vi "Definition.vi"(11 "User":refnum<class "User.lvclass">) -> (2 "Entity Definition":refnum<class "Type.lvclass">[](array[class]))   [LabVIEW 2022 SP3, in "Conditum-Example.lvlib" / "User.lvclass"]
uses:
  User.lvclass
  Conditum/Columns/Type/Type.lvclass
  Conditum/Columns/String/String.lvclass
  C:/dev/lv/illuminated-g/lv-conditum/Conditum/Columns/Type/Type.lvclass
  Conditum/Columns/Integer/Integer.lvclass
  Conditum/Columns/Timestamp/Timestamp.lvclass
  Conditum/Columns/Boolean/Boolean.lvclass
  User.lvclass/User.ctl
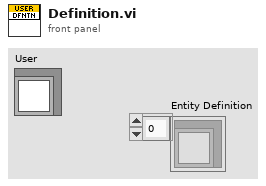
[diagram p1: front panel]
types:
  T1 = cluster{"Username":refnum<class "String.lvclass">, "Password":refnum<class "String.lvclass">, "Score":refnum<class "Integer.lvclass">, "Email":refnum<class "String.lvclass">, "Joined":refnum<class "Timestamp.lvclass">, "Has Logged In":refnum<class "Boolean.lvclass">, "Created Games":refnum<class "Entity Collection.lvclass">, "Joined Games":refnum<class "Entity Collection.lvclass">}
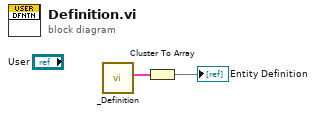
[diagram p0: block diagram]
diagram:
  n1 = call "_Definition.vi"() -> ("Definition"=w2:T1)  [unwired: 11 in]
  n2 = Cluster To Array(cluster=w2) -> (array=→"Entity Definition":refnum<class "Type.lvclass">[])
